vi "Set Window Z-Position (hwnd).vi"(8 "error in (no error)":errorcluster, 9 "Activate? (F)":bool, 10 "Z-Order Position":i16(ring) items=["Not Topmost", "Topmost", "Top", "Bottom"], 11 "HWnd":u32) -> (0 "error out":errorcluster, 3 "HWnd Out":u32)   [LabVIEW 2011]
doc: "-------------\nDeveloped by Brian Hoover (hooovahh)"
uses:
  User32.dll
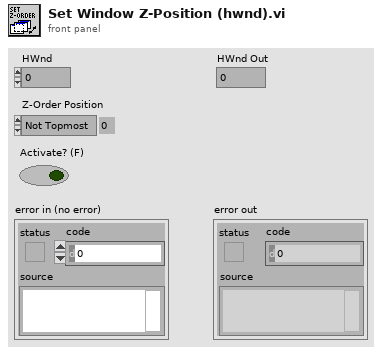
[diagram p1: front panel]
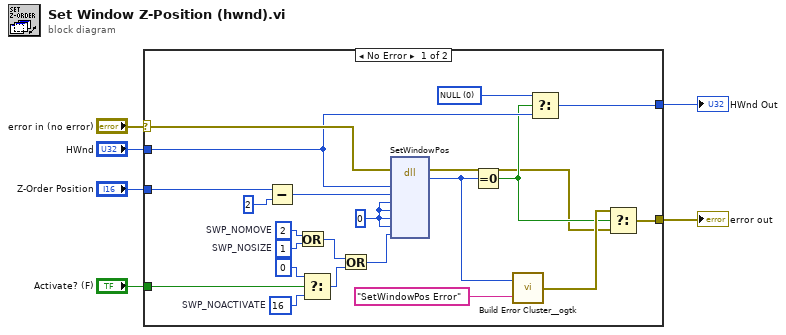
[diagram p0: block diagram]
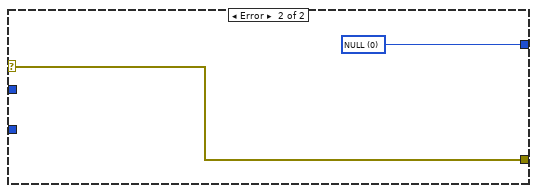
[diagram p2: hidden frame]
diagram:
  n1 = case shown="No Error" "error in (no error)" {
    selector: "error in (no error)" -> [w16 w30]
    tunnel: [w7 w30] -> w3
    tunnel: [w18 w29] -> w5
    tunnel: "HWnd" -> [w13 _]
    tunnel: "Activate? (F)" -> [w15 _]
    tunnel: "Z-Order Position" -> [w14 _]
    frame No Error {
      w17 = u32 0 items=["NULL"]
      w21 = u32 2  # SWP_NOMOVE
      w22 = u32 1  # SWP_NOSIZE
      w23 = u32 16  # SWP_NOACTIVATE
      w28 = 0
      n2 = Subtract(x=w14, y=i16 2) -> (x-y=w20:i16)
      n3 = Or(x=w21, y=w22) -> (x .or. y?=w26:u32)
      n4 = Select(t=u32 0, s=w15, f=w23) -> (s? t:f=w25:u32)
      n5 = Or(x=w26, y=w25) -> (x .or. y?=w27:u32)
      n6 = dll-call lib="USER32.DLL" fn="SetWindowPos"(error in=w16, "hWnd"=w13, "hWndInsertAfter"=w20, "left"=w28, "top"=w28, "width"=w28, "height"=w28, "fuFlags"=w27) -> (error out=w8:errorcluster, "error"=w11:i32)  [unwired: 8 in, 2 out]
      n7 = Equal To 0?(x=w11) -> (x = 0?=w9:bool)
      n8 = call <userlib>:"Build Error Cluster__ogtk.vi"("String to Prepend to source (\"\")"="SetWindowPos Error" ("String to Prepend to source (\"\")"), "code"=w11) -> ("error out"=w10:errorcluster)
      n9 = Select(t=w17, s=w9, f=w13) -> (s? t:f=w18:u32)
      n10 = Select(t=w10, s=w9, f=w8) -> (s? t:f=w7:errorcluster)
    }
    frame Error {
      w29 = u32 0 items=["NULL"]
    }
  }
  "HWnd Out" <- w5
  "error out" <- w3
